vi "BuildLogFilter.vi"(3 "FilterContents":T1) -> (1 "FilterString":string)   [LabVIEW 2013]
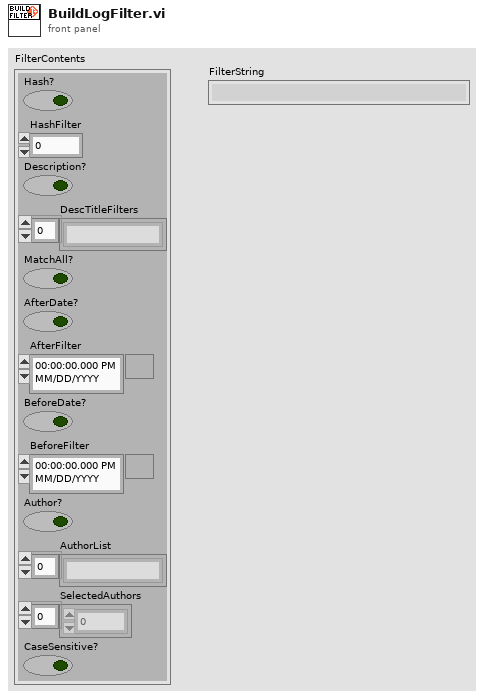
[diagram p1: front panel]
types:
  T1 = cluster{"Hash?":bool, "HashFilter":u64, "Description?":bool, "DescTitleFilters":string[], "MatchAll?":bool, "AfterDate?":bool, "AfterFilter":timestamp, "BeforeDate?":bool, "BeforeFilter":timestamp, "Author?":bool, "AuthorList":string[], "SelectedAuthors":i32[], "CaseSensitive?":bool}
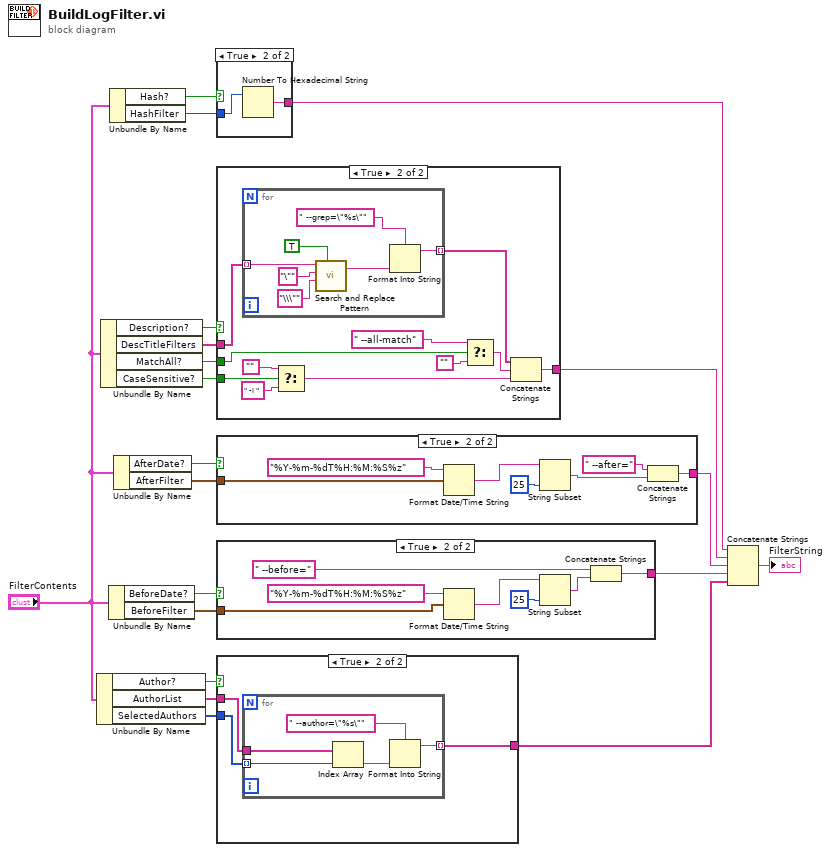
[diagram p0: block diagram]
diagram:
  n1 = Unbundle By Name("FilterContents") -> ("Author?"=w3:bool, "AuthorList"=w4:string[], "SelectedAuthors"=w2:i32[])
  n2 = Unbundle By Name("FilterContents") -> ("Description?"=w12:bool, "DescTitleFilters"=w11:string[], "MatchAll?"=w10:bool, "CaseSensitive?"=w1:bool)
  n3 = Unbundle By Name("FilterContents") -> ("BeforeDate?"=w9:bool, "BeforeFilter"=w8:timestamp)
  n4 = Unbundle By Name("FilterContents") -> ("Hash?"=w14:bool, "HashFilter"=w13:u64)
  n5 = Unbundle By Name("FilterContents") -> ("AfterDate?"=w7:bool, "AfterFilter"=w6:timestamp)
  n6 = case shown="True" w14 {
    tunnel: [_ w22] -> w15
    tunnel: w13 -> [_ w21]
    frame False {
    }
    frame True {
      n7 = Number To Hexadecimal String(2:w21) -> (0:w22:string)  [unwired: 1 in]
    }
  }
  n8 = case shown="True" w12 {
    tunnel: [_ w29] -> w16
    tunnel: w10 -> [_ w28]
    tunnel: w11 -> [_ w27]
    tunnel: w1 -> [_ w26]
    frame False {
    }
    frame True {
      n9 = for {
        tunnel: w27 -> [w39] mode=indexing
        tunnel: [w34] -> w33 mode=indexing
        n10 = call <vilib>:"Search and Replace Pattern.vi"("string"=w39, "regular expression (\"\")"="\"" ("regular expression (\"\")"), "replace string (\"\")"="\\\"" ("replace string (\"\")"), "replace all? (F)"=TRUE) -> ("result string"=w37:string)  [unwired: 1 in, 1 out]
        n11 = Format Into String(format string=" --grep=\"%s\"", w37) -> (resulting string=w34:string)  [unwired: 2 in, 1 out]
      }
      n12 = Select(t="", s=w26, f=" -i ") -> (s? t:f=w25:string)
      n13 = Select(t=" --all-match", s=w28, f="") -> (s? t:f=w30:string)
      n14 = Concatenate Strings(w33, w30, w25) -> (w29:string)
    }
  }
  n15 = case shown="True" w7 {
    tunnel: [_ w43] -> w17
    tunnel: w6 -> [_ w44]
    frame False {
    }
    frame True {
      n16 = Format Date/Time String(time format string (%c)="%Y-%m-%dT%H:%M:%S%z", seconds (now)=w44) -> (date/time string=w46:string)  [unwired: 1 in]
      n17 = String Subset(string=w46, length (rest)=25 ("length (rest)")) -> (substring=w42:string)  [unwired: 1 in]
      n18 = Concatenate Strings(" --after=", w42) -> (w43:string)
    }
  }
  n19 = case shown="True" w9 {
    tunnel: [_ w50] -> w18
    tunnel: w8 -> [_ w51]
    frame False {
    }
    frame True {
      n20 = Format Date/Time String(time format string (%c)="%Y-%m-%dT%H:%M:%S%z", seconds (now)=w51) -> (date/time string=w53:string)  [unwired: 1 in]
      n21 = String Subset(string=w53, length (rest)=25 ("length (rest)")) -> (substring=w49:string)  [unwired: 1 in]
      n22 = Concatenate Strings(" --before=", w49) -> (w50:string)
    }
  }
  n23 = case shown="True" w3 {
    tunnel: [_ w57] -> w19
    tunnel: w2 -> [_ w56]
    tunnel: w4 -> [_ w55]
    frame False {
    }
    frame True {
      n24 = for {
        tunnel: w56 -> [w62] mode=indexing
        tunnel: w55 -> [w61]
        tunnel: [w58] -> w57 mode=indexing
        n25 = Index Array(array=w61, index=w62) -> (element=w59:string)
        n26 = Format Into String(format string=" --author=\"%s\"", w59) -> (resulting string=w58:string)  [unwired: 2 in, 1 out]
      }
    }
  }
  n27 = Concatenate Strings(w15, w16, w17, w18, w19) -> (→"FilterString":string)
